vi "test malleable float to bytes.vi"() -> ()   [LabVIEW 2018, in "LV-Julia_ZMQ-Roundtrip_lib.lvlib"]
uses:
  LV-Julia_ZMQ-Roundtrip_lib.lvlib
  Bindata description.ctl
  64f9d793-bb93-41fe-8723-108ede85f934.vi
  64f9d793-bb93-41fe-8723-108ede85f934.vi/d1fb6aba-3f78-4c1e-843e-cfd750192278.vi
  64f9d793-bb93-41fe-8723-108ede85f934.vi/d1fb6aba-3f78-4c1e-843e-cfd750192278.vi/d0edf5b9-169c-4706-a44b-b3e5ad36fb4d.vi
  64f9d793-bb93-41fe-8723-108ede85f934.vi/d1fb6aba-3f78-4c1e-843e-cfd750192278.vi/d0edf5b9-169c-4706-a44b-b3e5ad36fb4d.vi/e6d19cc3-5c30-4a4d-9aeb-b238db6697dd.vi
  check ID validity.vi
panel:
  out "Bindata & descr out":cluster{"bindata_descr":T1[], "bindata":u8[]}
  out "error out":errorcluster
  in  "Tag":string
  out "flattened array":dbl[](array[numeric])
  in  "Array":sgl[][](array[numeric])
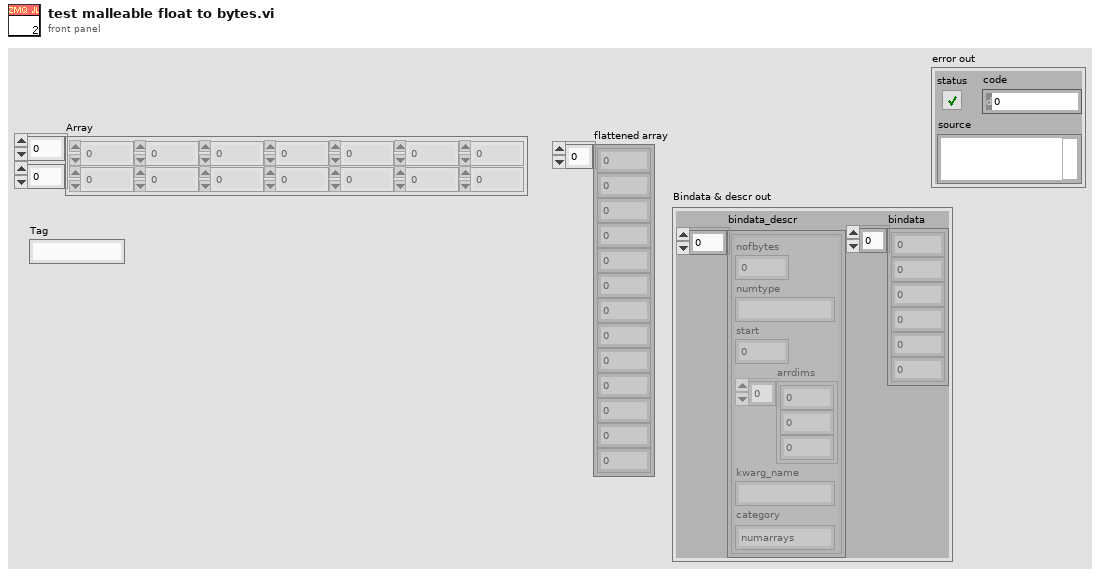
[diagram p1: front panel]
types:
  T1 = typedef "LV-Julia_ZMQ-Roundtrip_lib.lvlib/Bindata description.ctl" = cluster{"nofbytes":i32, "numtype":string, "start":i32, "arrdims":i32[], "kwarg_name":string, "category":string}
  T2 = typedef "Bindata&description.ctl" = cluster{"bindata_descr":T1[], "bindata":u8[]}
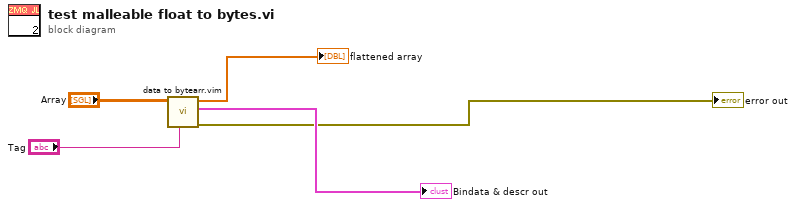
[diagram p0: block diagram]
diagram:
  n1 = call "data to bytearr.vim"("kwarg_name"="Tag", "data in"="Array") -> ("error out"=→"error out":errorcluster, "Bindata & descr out"=→"Bindata & descr out":T2, "flattened data out"=→"flattened array":sgl[])  [unwired: 7 in]
